vi "DSP_GetVersion.vi"(4 "error in (no error)":errorcluster, 7 "Board Handle":u64) -> (0 "error out":errorcluster, 1 "Minor":u32, 2 "Major":u32, 3 "Board Handle Out":u64)   [LabVIEW 2009]
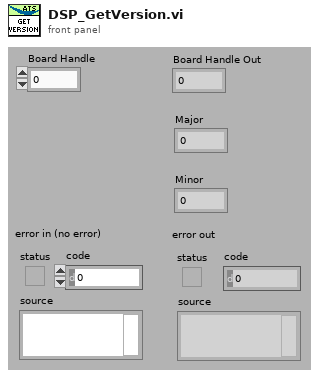
[diagram p1: front panel]
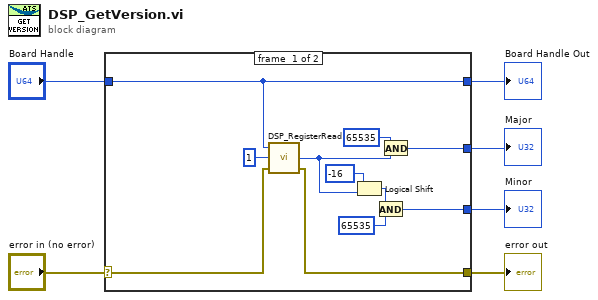
[diagram p0: block diagram]
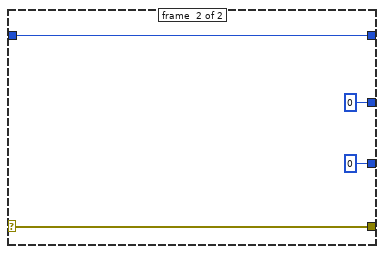
[diagram p2: hidden frame]
diagram:
  n1 = case shown="No Error" "error in (no error)" {
    selector: "error in (no error)" -> [w16 w21]
    tunnel: [w15 w21] -> w5
    tunnel: [w17 w20] -> w4
    tunnel: "Board Handle" -> [w17 w20]
    tunnel: [w12 u32 0] -> w1
    tunnel: [w7 u32 0] -> w2
    frame #0 {
      n2 = call "DSP_RegisterRead.vi"("error in (no error)"=w16, "Offset"=u32 1, "Board Handle"=w17) -> ("error out"=w15:errorcluster, "Value"=w10:u32)  [unwired: 1 out]
      n3 = Logical Shift(y=-16, x=w10) -> (x << y=w9:u32)
      n4 = And(x=w9, y=u32 65535) -> (x .and. y?=w7:u32)
      n5 = And(x=u32 65535, y=w10) -> (x .and. y?=w12:u32)
    }
    frame #1 {
    }
  }
  "Board Handle Out" <- w4
  "error out" <- w5
  "Minor" <- w2
  "Major" <- w1
